vi "tls read up to clrf.vi"(7 "max size":i32, 8 "error in":errorcluster, 9 "timeout ms":i32, 10 "buffer in":string, 11 "lvlibretls connection in":refnum<class "lvlibretls connection.lvclass">) -> (0 "error out":errorcluster, 2 "buffer out":string, 3 "line out":string)   [LabVIEW 2016, in "TLS HTTP server.lvclass"]
uses:
  TLS HTTP server.lvclass
  lvlibtls/socket connection/lvlibretls connection.lvclass
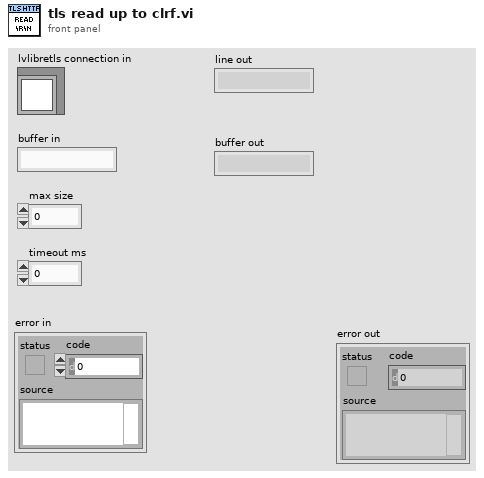
[diagram p1: front panel]
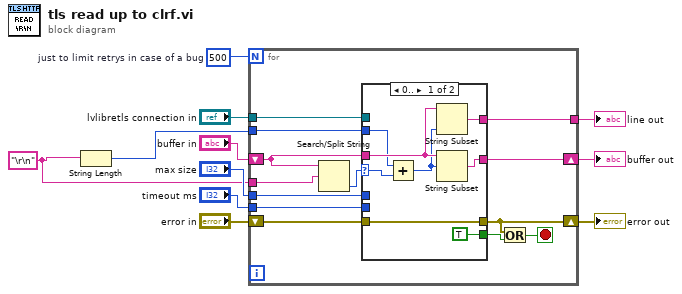
[diagram p0: block diagram]
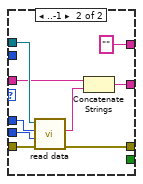
[diagram p2: hidden frame]
diagram:
  w2 = "\r\n" ("search string/char (-)")
  w5 = 500  # just to limit retrys in case of a bug
  n1 = String Length(string=w2) -> (length=w1:i32)
  n2 = for {
    N: w5 -> [_]
    tunnel: "lvlibretls connection in" -> [w24]
    tunnel: [w20] -> w3
    shift-right: [w21] -> w4
    shift-left: "buffer in" -> [w14]
    shift-right: [w18] -> w8
    shift-left: "error in" -> [w23]
    tunnel: "max size" -> [w16]
    tunnel: "timeout ms" -> [w15]
    tunnel: w2 -> [w13]
    tunnel: w1 -> [w12]
    stop <- w19 stop-if-true
    n3 = Search/Split String(string=w14, search string/char (-)=w13) -> (offset of match=w22:i32)  [unwired: 1 in, 2 out]
    n4 = case shown="0.." w22 {
      selector: w22 -> [w27 _]
      tunnel: w24 -> [_ w41]
      tunnel: w23 -> [w32 w40]
      tunnel: [w32 w39] -> w18
      tunnel: [w28 w37] -> w21
      tunnel: [w29 "" ("data in")] -> w20
      tunnel: [TRUE _] -> w17
      tunnel: w16 -> [_ w35]
      tunnel: w15 -> [_ w34]
      tunnel: w14 -> [w30 w33]
      tunnel: w12 -> [w25 _]
      frame 0.. {
        n5 = Add(x=w25, y=w27) -> (x+y=w26:i32)
        n6 = String Subset(string=w30, length (rest)=w26) -> (substring=w29:string)  [unwired: 1 in]
        n7 = String Subset(string=w30, offset (0)=w26) -> (substring=w28:string)  [unwired: 1 in]
      }
      frame ..-1 {
        n8 = call "read data.vi"("error in"=w40, "timeout"=w34, "max size"=w35, "lvlibretls connection in"=w41) -> ("error out"=w39:errorcluster, "data"=w38:string)  [unwired: 5 in, 1 out]
        n9 = Concatenate Strings(w33, w38) -> (w37:string)
      }
    }
    n10 = Or(x=w18, y=w17) -> (x .or. y?=w19:bool)
  }
  "buffer out" <- w4
  "line out" <- w3
  "error out" <- w8
